vi "ShouldWeChangeRegime.vi"(10 "Desired Sailing Regime":T1, 11 "Current Sailing Regime":T1) -> (3 "ShouldWeChangeRegime?":bool)   [LabVIEW 2013]
doc: "Determines whether the boat should change regimes, simply by checking the boat regime against the desired regime. It then determines which regime we should enter based on our desired end state.\n\nCurrently the logic is dead-simple, and doesn't necessarily require a VI, but if in the future we might want to change regimes for more complex reasons, this is where that logic would go.\n\nEric Schneider"
uses:
  Data/TypeDefs/Sailing Regimes.ctl
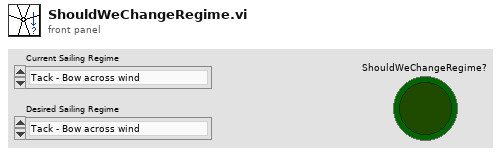
[diagram p1: front panel]
types:
  T1 = typedef "Sailing Regimes.ctl" = enum16{"Tack - Bow across wind", "Upwind - Port Tack", "Turn between Upwind/Reach - Port Tack", "Reach - Port Tack", "Turn between Reach/Run - Port Tack", "Run - Port Tack", "Jibe - Stern across wind", "Run - Starboard Tack", "Turn between Reach/Run - Starboard Tack", "Reach - Starboard Tack", "Turn between Upwind/Reach - Starboard Tack", "Upwind - Starboard Tack"}
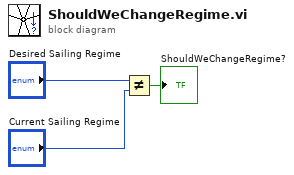
[diagram p0: block diagram]
diagram:
  n1 = Not Equal?(x="Desired Sailing Regime", y="Current Sailing Regime") -> (x != y?=→"ShouldWeChangeRegime?":bool)
